vi "AddConstantResistance.vi"(0 "deviceName":string, 1 "channel":u8, 2 "repeats":u16=1, 3 "resistance":sgl, 4 "samplingInterval":sgl, 5 "maxDuration":sgl, 6 "minVoltage":sgl=-inf, 7 "error in (no error)":errorcluster, 8 "isMinimumVoltageVsOCP":bool, 9 "maxVoltage":sgl=inf, 10 "isMaximumVoltageVsOCP":bool, 11 "maxCurrent":sgl=inf, 12 "minCurrent":sgl=-inf, 13 "maxCapacity":sgl=inf) -> (27 "error out":errorcluster)   [LabVIEW 2018]
doc: "EXPORT void AisAddConstantResistance(const char* deviceName, uint8_t channel, uint16_t repeats, float resistance, float samplingInterval, float maxDuration, float minVoltage, bool isMinimumVoltageVsOCP, float maxVoltage, bool isMaximumVoltageVsOCP, float maxCurrent, float minCurrent, float maxCapacity);"
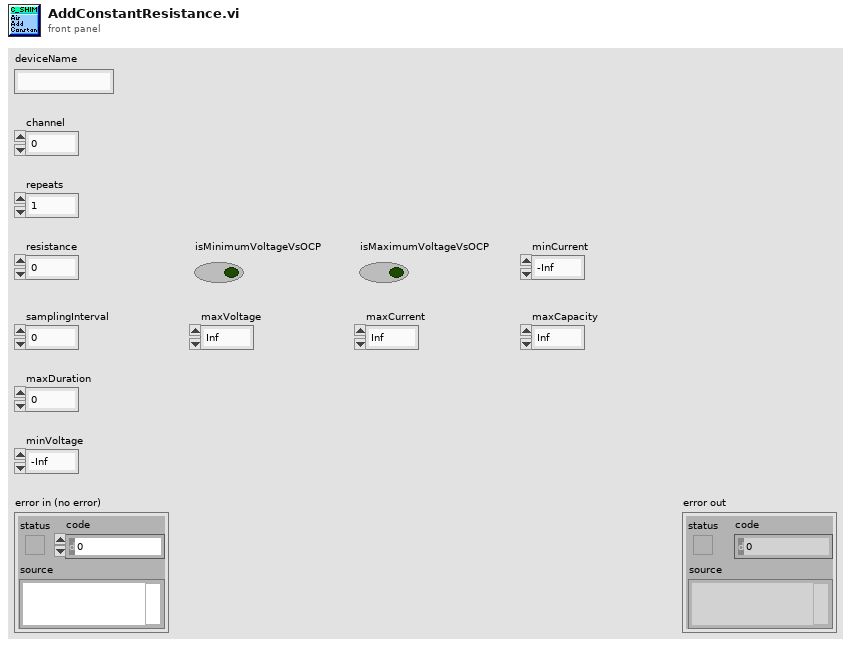
[diagram p1: front panel]
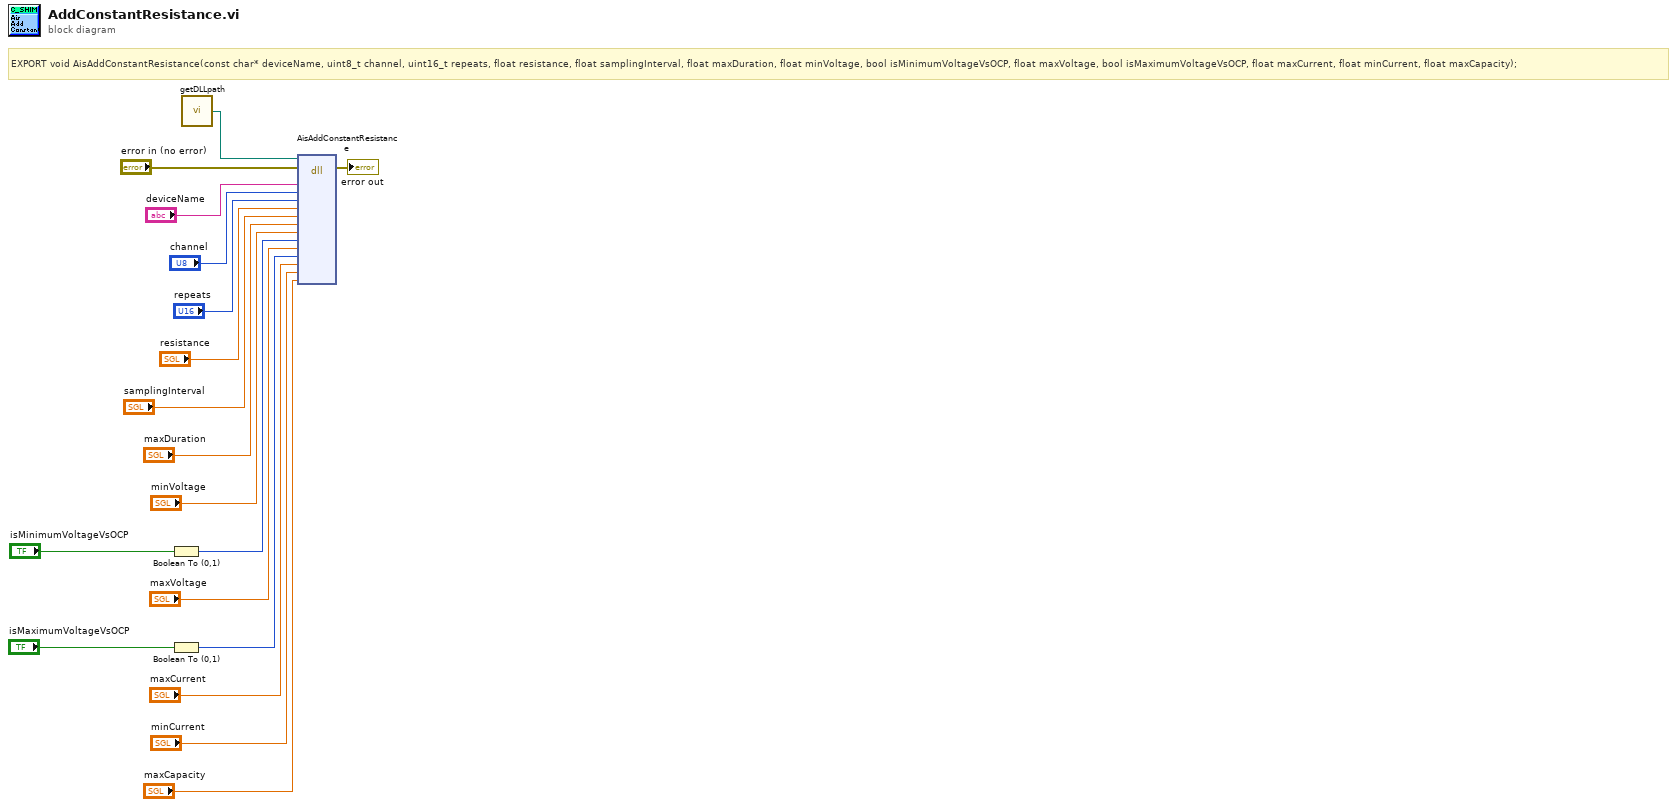
[diagram p0: block diagram]
diagram:
  # "EXPORT void AisAddConstantResistance(const char* deviceName, uint8_t channel, uint16_t repeats, float resistance, float samplingInterval, float maxDuration, float minVoltage, bool isMinimumVoltageVsOCP, float maxVoltage, bool isMaximumVoltageVsOCP, float maxCurrent, float minCurrent, float maxCapacity);"
  n1 = Boolean To (0,1)(Boolean="isMinimumVoltageVsOCP") -> (0, 1=w10:i16)
  n2 = Boolean To (0,1)(Boolean="isMaximumVoltageVsOCP") -> (0, 1=w7:i16)
  n3 = call "getDLLpath.vi"() -> ("DLL_Path"=w1:path)
  n4 = dll-call lib="?" fn="AisAddConstantResistance"(path in=w1, error in="error in (no error)", "deviceName"="deviceName", "channel"="channel", "repeats"="repeats", "resistance"="resistance", "samplingInterval"="samplingInterval", "maxDuration"="maxDuration", "minVoltage"="minVoltage", "isMinimumVoltageVsOCP"=w10, "maxVoltage"="maxVoltage", "isMaximumVoltageVsOCP"=w7, "maxCurrent"="maxCurrent", "minCurrent"="minCurrent", "maxCapacity"="maxCapacity") -> (error out=→"error out":errorcluster)  [unwired: 15 in, 1 out]
